vi "Read.vi"(8 "error in (no error)":errorcluster, 11 "Reset Var Command Config in":refnum<class "Reset Var Command Config.lvclass">) -> (0 "error out":errorcluster, 2 "Names":string[](array[string]), 3 "Reset Var Command Config out":refnum<class "Reset Var Command Config.lvclass">)   [LabVIEW 2020, in "VolatusSeqConfig.lvlib" / "Reset Var Command Config.lvclass"]
uses:
  Reset Var Command Config.lvclass
  Reset Var Command Config.lvclass/Reset Var Command Config.ctl
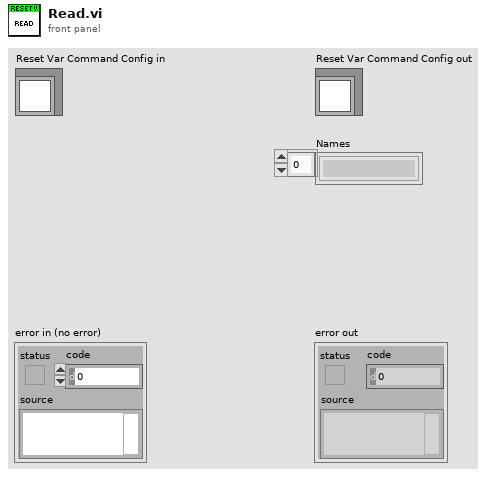
[diagram p1: front panel]
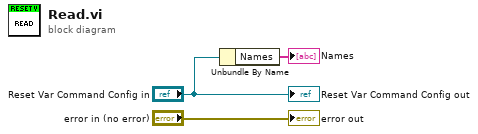
[diagram p0: block diagram]
diagram:
  n1 = Unbundle By Name("Reset Var Command Config in") -> ("Names"=→"Names":string[])
  "error out" <- "error in (no error)"
  "Reset Var Command Config out" <- "Reset Var Command Config in"
